vi "Software Version ermitteln.vi"(8 "error in (no error)":errorcluster caption="Fehler (Eingang, kein Fehler)", 10 "Istwerte":u16[](array[numeric]), 11 "Steuerung PNS Eingang":refnum<class "Steuerung PNS.lvclass">) -> (0 "error out":errorcluster caption="Fehler (Ausgang)", 2 "SoftWare Vresion":string, 3 "Steuerung PNS Ausgang":refnum<class "Steuerung PNS.lvclass">)   [LabVIEW 2020, in "Steuerung PNS.lvclass"]
uses:
  Steuerung PNS.lvclass
  Steuerung PNS.lvclass/Steuerung PNS.ctl
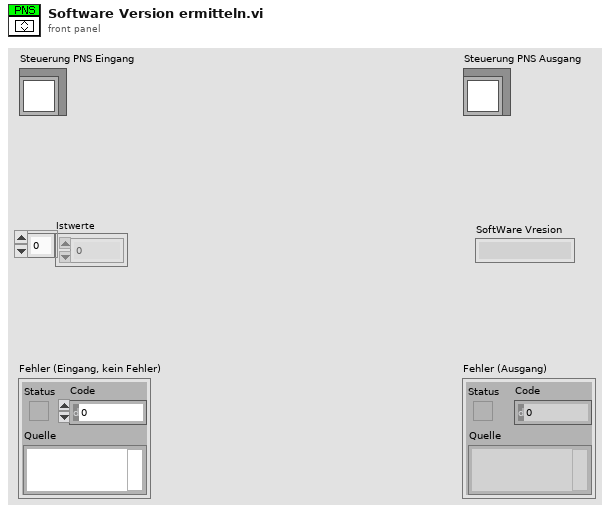
[diagram p1: front panel]
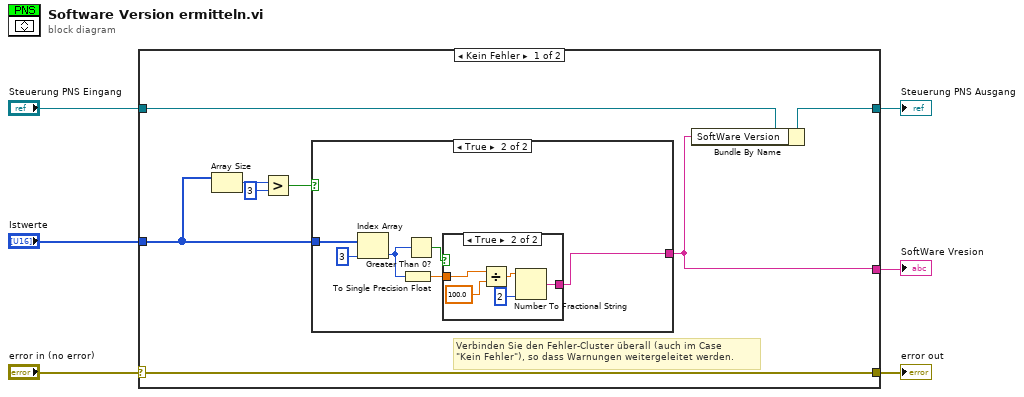
[diagram p0: block diagram]
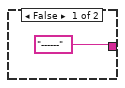
[diagram p2: hidden frame]
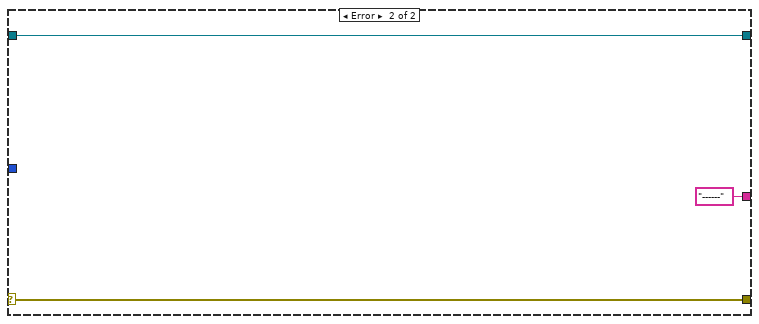
[diagram p4: hidden frame]
diagram:
  n1 = case shown="Kein Fehler" "error in (no error)" {
    selector: "error in (no error)" -> [w14 w29]
    tunnel: [w14 w29] -> w5
    tunnel: [w12 w28] -> w3
    tunnel: "Steuerung PNS Eingang" -> [w13 w28]
    tunnel: "Istwerte" -> [w10 _]
    tunnel: [w11 "------"] -> w1
    frame No Error {
      # "Verbinden Sie den Fehler-Cluster überall (auch im Case\n\"Kein Fehler\"), so dass Warnungen weitergeleitet werden."
      n2 = Array Size(array=w10) -> (size(s)=w9:i32)
      n3 = Greater?(x=w9, y=3) -> (0:w7:bool)
      n4 = case shown="True" w7 {
        tunnel: ["------" w19] -> w11
        tunnel: w10 -> [_ w20]
        frame False {
        }
        frame True {
          n5 = Index Array(array=w20, index=3 ("Index")) -> (element=w18:u16)
          n6 = To Single Precision Float(number=w18) -> (single precision float=w16:sgl)
          n7 = Greater Than 0?(x=w18) -> (x > 0?=w17:bool)
          n8 = case shown="True" w17 {
            tunnel: w16 -> [_ w25]
            tunnel: [_ w26] -> w19
            frame False {
            }
            frame True {
              n9 = Divide(x=w25, y=sgl 100.0) -> (x/y=w24:sgl)
              n10 = Number To Fractional String(number=w24, precision (6)=i16 2 ("Genauigkeit (6)")) -> (F-format string=w26:string)  [unwired: 2 in]
            }
          }
        }
      }
      n11 = Bundle By Name(cluster=w13, "SoftWare Version"=w11) -> (w12:refnum<class "Steuerung PNS.lvclass">)
    }
    frame Error {
    }
  }
  "error out" <- w5
  "Steuerung PNS Ausgang" <- w3
  "SoftWare Vresion" <- w1
